vi "Simulated gated signals.vi"() -> ()   [LabVIEW 2022 SP3]
doc: "Performs real-time Joint Time Frequency Analysis (JTFA) using Point By Point STFT. The signal is simulated by a sine wave plus Gaussian noise."
uses:
  <vilib>/measure/mamon.llb/Waveform Peak Detection for N Chan.vi
  <vilib>/measure/NI_MAPro.lvlib
  <vilib>/gmath/NI_Gmath.lvlib
  <vilib>/Analysis/NI_AALBase.lvlib
panel:
  out "sampling frequency":dbl=16000.0
  out "BPM":dbl=260.6047910019081
  out "standard deviation":dbl=0.007320347822328487 format="%.4f"
  out "mean":dbl=0.23023367977744008 format="%.3f"
  out "Heart rates":dbl[](array[numeric])=[0.0, 0.23739526238057532, 0.21927218547308347, 0.22913219297822318, 0.2288319629419665, 0.2365367951133519]
  out "Waveform Graph 3":dynamicdata(graph)=[{"t0"=timestamp(0 s since 1904-01-01), "dt"=0.004, "Y"=array[365 elements], "attributes"=variant("NI_ChannelName"=variant(string "Filtered"))}]
  out "Array 4":i32[](array[numeric])=[1, 1, 1, 1, 1, 1, 1, 1, 1, 1, 0, 0, 0, 0, 0, 0, 0, 0, 1, 0, 0, 0, 0, 0, 0, 0, 0, 0, 0, 0, 0, 2, 0, 3, 4, 2, 5, 6, 3, 5, 7, 6, 7, 6, 6, 4, 5, 4, 6, 4, 4, 2, 3, 4, 2, 2, 1, 2, 1, 1, 1, 0, 0, 0, 0, 0, 0, 0, 0, 0, 0, 0, 0, 0, 0, 0, 0, 0, 0, 0, 0, 1, 1, 1, 1, 0, 0, 0, 1, 4, 2, 5, 4, 5, 4, 5, 3, 7, 5, 7, 5, 6, 5, 6, 5, 5, 5, 5, 6, 4, 2, 4, 2, 2, 2, 2, 1, 2, 1, 1, 1, 1, 1, 0, 0, 0, 0, 0, 1, 0, 1, 0, 0, 1, 0, 0, 0, 0, 0, 0, 0, 1, 0, 0, 1, 2, 2, 4, 6, 6, 6, 4, 8, 7, 5, 8, 5, 4, 5, 7, 6, 7, 5, 5, 5, 4, 4, 3, 3, 4, 3, 3, 1, 1, 1, 1, 1, 0, 1, 0, 0, 0, 0, 1, 0, 0, 0, 0, 1, 0, 0, 0, 0, 0, 0, 0, 0, 0, 1, 0, 0, 0, 3, 4, 4, 6, 6, 5, 6, 8, 8, 7, 6, 6, 7, 6, 6, 5, 7, 6, 6, 6, 5, 3, 4, 5, 3, 3, 2, 1, 1, 1, 1, 1, 0, 1, 0, 0, 1, 0, 0, 0, 0, 0, 0, 1, 0, 1, 0, 0, 1, 0, 1, 0, 1, 0, 1, 0, 1, 0, 2, 2, 3, 1, 4, 6, 5, 3, 5, 6, 4, 3, 3, 3, 3, 4, 3, 2, 2, 3, 4, 2, 2, 2, 2, 2, 2, 1, 1, 1, 1, 1, 1, 1, 1, 1, 1, 1, 1, 0, 0, 0, 1, 0, 0, 0, 0, 0, 0, 2, 0, 0, 0, 0, 0, 0, 1, 3, 3, 4, 5, 2, 4, 6, 4, 4, 5, 6, 6, 5, 6, 6, 6, 6, 6, 4, 5, 4, 2, 4, 3, 4, 2, 1, 1, 1, 1, 0, 1, 1, 1, 0, 0, 0, 1, 0, 0, 0, 0, 0, 0, 1, 0, 0, 1]
  out "Width 2":i32=365
  in  "time-freq config":cluster{"power of 2":bool, "Nyquist":bool}
  in  "Threshold":dbl=5.0
  in  "Width":i32=4
  in  "stop 2":bool
  out "Number of samples":i32=23336
  out "Extracted":dynamicdata(graph)=[{"t0"=timestamp(1.3140625000000001 s since 1904-01-01), "dt"=6.25e-05, "Y"=array[23336 elements], "attributes"=variant("NI_ChannelName"=variant(string "Dev1/ai0 (Extracted)"), "NI_ExpIsRelativeTime"=variant(bool TRUE), "NI_ExpStartTimeStamp"=variant(timestamp timestamp(3271175784.421062 s since 1904-01-01)), "NI_ExpTimeStamp"=variant(timestamp timestamp(3271175788.8760614 s since 1904-01-01)), "NI_ExpXDimension"=variant(string "t"), "NI_OriginalChannelName"=variant(string "Dev1/ai0"))}] caption="Signals"
  in  "process data":bool
  in  "time-freq sampling":cluster{"time steps":i32, "freq bins":i32}={"time steps"=64, "freq bins"=128} {"freq bins" format="%0.0f"}
  in  "window info":cluster{"type":u32, "window length":u32}={"type"=2, "window length"=128} {"window length" format="%0.0f"; "type" format="%0.0f"}
  out "Waveform Graph 2":waveform(dbl)(graph)={"t0"=timestamp(0 s since 1904-01-01), "dt"=0.004, "Y"=array[365 elements]}
  out "Locations":cluster{"Locations":dbl[]}[](array[cluster])=[{"Locations"=[49.01745339243051, 108.36626898757434, 163.1843153558452, 220.467363600401, 277.6753543358926, 336.8095531142306]}] {"Locations" format="%.2p"}
  out "Amplitudes":cluster{"Amplitudes":dbl[]}[](array[cluster])=[{"Amplitudes"=[82.38140614123277]}, {"Amplitudes"=[23.103240542422952]}, {"Amplitudes"=[179.84302922359947]}, {"Amplitudes"=[69.20602969118777]}, {"Amplitudes"=[166.80882400642417]}, {"Amplitudes"=[77.52276422393723]}, {"Amplitudes"=[21.4640593868428]}, {"Amplitudes"=[20.107049640024623]}, {"Amplitudes"=[8.747151960239117]}, {"Amplitudes"=[22.2070032831398]}, {"Amplitudes"=[]}, {"Amplitudes"=[]}, {"Amplitudes"=[]}, {"Amplitudes"=[]}, {"Amplitudes"=[]}, {"Amplitudes"=[]}, {"Amplitudes"=[]}, {"Amplitudes"=[]}, {"Amplitudes"=[5.038436740788092]}, {"Amplitudes"=[]}, {"Amplitudes"=[]}, {"Amplitudes"=[]}, {"Amplitudes"=[]}, {"Amplitudes"=[]}, {"Amplitudes"=[]}, {"Amplitudes"=[]}, {"Amplitudes"=[]}, {"Amplitudes"=[]}, {"Amplitudes"=[]}, {"Amplitudes"=[]}, {"Amplitudes"=[]}, {"Amplitudes"=[22.842667263708673, 6.3391147998422825]}, {"Amplitudes"=[]}, {"Amplitudes"=[24.87960791496652, 18.099361302359405, 11.032350413832436]}, {"Amplitudes"=[32.15025039562714, 13.922752510400683, 7.537223901883069, 8.901460877167851]}, {"Amplitudes"=[6.919633956075483, 6.805974509190123]}, {"Amplitudes"=[9.291208559626742, 9.83940570113674, 19.712031302498918, 10.262114635729274, 16.148451130689434]}, {"Amplitudes"=[58.61965660372665, 9.272847341081285, 10.229585203806352, 8.33485828928211, 8.53822283822932, 10.363752661085321]}, {"Amplitudes"=[32.99317191422573, 25.184044683933838, 6.176018204109812]}, {"Amplitudes"=[24.784936643849996, 11.180097278969077, 10.426571385559898, 9.147862049386452, 5.3056033973289445]}, {"Amplitudes"=[28.86732717209763, 57.63574400772855, 9.936407211583475, 15.352865769442293, 7.430357498420502, 9.113919835956231, 5.758941008482342]}, {"Amplitudes"=[30.501710958611454, 9.983123212214235, 49.565628988940404, 15.957520448688324, 5.142299425348082, 5.542245542198177]}, {"Amplitudes"=[13.584188049747981, 21.738357840547337, 21.353114728112995, 19.064944754501603, 12.767713772677945, 5.8155103082985375, 12.38997676581007]}, {"Amplitudes"=[19.17611366053601, 18.03811348206983, 21.946319425374636, 29.131558149158767, 7.854839251223176, 7.587917409227231]}, {"Amplitudes"=[26.251064738468205, 22.32439049471829, 13.733976720916365, 14.284625689843542, 11.06250138130756, 29.699723502437603]}, {"Amplitudes"=[13.92238514317977, 7.02343083135868, 95.53112318708045, 11.003700676197488]}, {"Amplitudes"=[75.27576626556457, 108.6469533115197, 46.189476972060085, 6.657679907425096, 6.508395743341386]}, {"Amplitudes"=[38.93368826176039, 22.453719389339394, 15.70774563803036, 25.85362047641387]}, {"Amplitudes"=[16.43990619327277, 11.31756210221035, 24.319042387903707, 22.55410151565015, 17.576151247289495, 6.909780980309922]}, {"Amplitudes"=[38.642716598694676, 68.69914689572425, 15.77436441173343, 17.57003043557135]}, {"Amplitudes"=[45.619636519793985, 66.77776746865493, 27.414381321266774, 10.378734791849856]}, {"Amplitudes"=[31.52012443340925, 9.419069673822978]}, {"Amplitudes"=[14.282507680413168, 30.083275487465478, 10.56411972040232]}, {"Amplitudes"=[17.52357745400949, 39.06632267195957, 67.90378041221246, 7.03859185888409]}, {"Amplitudes"=[38.22382741700391, 78.81409489667777]}, {"Amplitudes"=[99.66718914407029, 39.26256050528829]}, {"Amplitudes"=[121.01146302765554]}, {"Amplitudes"=[43.06727266056416, 14.211732733807018]}, {"Amplitudes"=[334.0636434809306]}, {"Amplitudes"=[197.95811877505346]}, {"Amplitudes"=[7.628663545669674]}, {"Amplitudes"=[]}, {"Amplitudes"=[]}, {"Amplitudes"=[]}, {"Amplitudes"=[]}, {"Amplitudes"=[]}, {"Amplitudes"=[]}, {"Amplitudes"=[]}, {"Amplitudes"=[]}, {"Amplitudes"=[]}, {"Amplitudes"=[]}, {"Amplitudes"=[]}, {"Amplitudes"=[]}, {"Amplitudes"=[]}, {"Amplitudes"=[]}, {"Amplitudes"=[]}, {"Amplitudes"=[]}, {"Amplitudes"=[]}, {"Amplitudes"=[]}, {"Amplitudes"=[]}, {"Amplitudes"=[]}, {"Amplitudes"=[38.02896888352999]}, {"Amplitudes"=[60.71594429484877]}, {"Amplitudes"=[77.864673975236]}, {"Amplitudes"=[86.75331398374871]}, {"Amplitudes"=[]}, {"Amplitudes"=[]}, {"Amplitudes"=[]}, {"Amplitudes"=[30.285694406280772]}, {"Amplitudes"=[6.70083506344839, 9.996184325043538, 13.161601140869823, 11.068127320638746]}, {"Amplitudes"=[12.179672839603471, 15.15864622255311]}, {"Amplitudes"=[6.757699919664426, 14.563558566945403, 30.0974793381078, 35.13852702699444, 11.82912775073785]}, {"Amplitudes"=[30.21628667420045, 37.19105776834435, 10.44811719015927, 5.979410571766171]}, {"Amplitudes"=[12.568666333491867, 10.525198573111078, 25.908754410806793, 23.480087021227384, 7.711006153248385]}, {"Amplitudes"=[8.069198985980876, 49.38285487269324, 16.54495588616374, 6.005677169490166]}, {"Amplitudes"=[9.974388294197606, 28.38980644929219, 12.125908243362064, 10.394406035302056, 12.273928645626906]}, {"Amplitudes"=[44.25850209386394, 45.36184860767733, 14.919613359784044]}, {"Amplitudes"=[25.551642802149477, 19.553635465036656, 47.25245815923574, 25.153362046593475, 14.160489368192284, 13.383198080728581, 15.616706212026298]}, {"Amplitudes"=[8.585910286384838, 49.15376283146787, 35.0730060764914, 19.924436039092853, 5.0061812311169795]}, {"Amplitudes"=[6.583257420688857, 6.2255192674828805, 45.69894868242657, 11.403330231694829, 23.57700544456967, 10.436565239964331, 11.383870447954372]}, {"Amplitudes"=[62.02127332764015, 33.96249128412671, 31.66759689025207, 23.0624840067356, 16.33642520284919]}, {"Amplitudes"=[34.415707375153936, 10.373696441976328, 26.156329918410478, 22.768141555256843, 10.750393432856006, 6.062207171974502]}, {"Amplitudes"=[32.48087650197277, 33.18602344776615, 17.890767174979935, 7.761315184410173, 5.7887068311030285]}, {"Amplitudes"=[37.083089931075314, 15.613396366499963, 12.051173949030618, 18.998380068120078, 5.577481300514407, 16.822493856755596]}, {"Amplitudes"=[116.412866314646, 47.39382629648723, 35.45067946475894, 8.848064961792382, 12.33559214796111]}, {"Amplitudes"=[36.55122432846308, 20.62731946396467, 19.524064296664893, 17.037236783177224, 12.75331545962354]}, {"Amplitudes"=[13.678435249173804, 17.977927437594456, 58.54736305377815, 37.905893287547244, 14.190662435858426]}, {"Amplitudes"=[19.7560860518155, 14.608744151622977, 14.997554396578456, 21.598462686694923, 6.803511160283876]}, {"Amplitudes"=[6.585864083905273, 16.35640196679662, 40.97026196636454, 5.74845196116436, 10.859839534328385, 26.432671751231265]}, {"Amplitudes"=[37.14491370258239, 8.786630443687102, 50.50402558068138, 6.9178735457692735]}, {"Amplitudes"=[43.03391314367019, 23.104668104550083]}, {"Amplitudes"=[19.23442411554904, 42.951474267999565, 8.326360458916051, 19.85487475354863]}, {"Amplitudes"=[67.38130875885368, 127.24575233366998]}, {"Amplitudes"=[230.59836703695711, 21.27374517334955]}, {"Amplitudes"=[117.60370625127554, 9.164920650883204]}, {"Amplitudes"=[34.48653974052241, 28.06721753602859]}, {"Amplitudes"=[97.08351402694935]}, {"Amplitudes"=[42.47704129034807, 11.196688692677348]}, {"Amplitudes"=[80.09104308548649]}, {"Amplitudes"=[17.024047125400102]}, {"Amplitudes"=[49.16287496060881]}, {"Amplitudes"=[37.874323635207055]}, {"Amplitudes"=[13.996901677633218]}, {"Amplitudes"=[]}, {"Amplitudes"=[]}, {"Amplitudes"=[]}, {"Amplitudes"=[]}, {"Amplitudes"=[]}, {"Amplitudes"=[21.059179416556383]}, {"Amplitudes"=[]}, {"Amplitudes"=[5.655247392917452]}, {"Amplitudes"=[]}, {"Amplitudes"=[]}, {"Amplitudes"=[7.566160612918716]}, {"Amplitudes"=[]}, {"Amplitudes"=[]}, {"Amplitudes"=[]}, {"Amplitudes"=[]}, {"Amplitudes"=[]}, {"Amplitudes"=[]}, {"Amplitudes"=[]}, {"Amplitudes"=[7.940747799708725]}, {"Amplitudes"=[]}, {"Amplitudes"=[]}, {"Amplitudes"=[171.89064010452762]}, {"Amplitudes"=[53.38985445160456, 47.20944180326978]}, {"Amplitudes"=[39.43321909539199, 41.42355004804408]}, {"Amplitudes"=[35.43003439390867, 39.79903190772515, 8.314447339982246, 5.522839392912958]}, {"Amplitudes"=[17.70458188715799, 22.27340772615113, 11.859423616096409, 16.196217369343895, 13.878592440001153, 9.367139271726463]}, {"Amplitudes"=[10.902753813737803, 51.224945091558666, 26.28363330510103, 12.775051212225032, 19.185592807108467, 16.064310141996202]}, {"Amplitudes"=[10.775132950480547, 9.837669766466332, 6.450044817928087, 40.14331590442509, 15.606677966367329, 5.604758984152606]}, {"Amplitudes"=[6.956894212125345, 36.49419940460505, 29.45502817761903, 8.942586285160438]}, {"Amplitudes"=[15.959514391389876, 18.853571112883863, 17.94415105779546, 38.525933539883226, 24.04328588184206, 21.273783492422787, 13.829695847414577, 7.0329830848447585]}, {"Amplitudes"=[19.739115058203684, 7.443389173941418, 59.547360360705206, 7.508154414957717, 7.263707742763704, 7.093406442203529, 13.645592171928815]}, {"Amplitudes"=[58.00433167997356, 66.44232976379686, 31.068545997989553, 7.732699625859007, 29.475986606683623]}, {"Amplitudes"=[20.029286291449644, 28.33111106014688, 8.409477614266663, 18.80578148132153, 21.171639700146116, 25.473492332663604, 7.755959491068256, 5.339663761530281]}, {"Amplitudes"=[48.57178655340573, 45.86566940589032, 33.80312552414865, 33.80004450551245, 5.5710069746768545]}, {"Amplitudes"=[33.80689208354685, 7.9078152784270115, 12.213787607759153, 8.29289788679703]}, {"Amplitudes"=[11.477744418191296, 50.28304189114041, 62.73404211139437, 9.263680695435566, 11.384540967823002]}, {"Amplitudes"=[20.993160472233647, 16.444118860252896, 16.553516223741497, 25.592202531125537, 5.470654244994138, 10.01144042489008, 9.484975090197048]}, {"Amplitudes"=[11.479156218631724, 14.712869975625633, 23.311470173881315, 30.955710724525687, 17.020590082910363, 26.38350872695788]}, {"Amplitudes"=[27.085772245284435, 11.746088084069942, 39.376986923391826, 24.5264042480838, 26.77428596744944, 5.6044046609893154, 5.298175841656865]}, {"Amplitudes"=[28.38274728899761, 76.88706276985069, 8.013736159658887, 8.38031009484177, 14.611102559246898]}, {"Amplitudes"=[76.77827122135417, 19.037720260357304, 9.60326338877064, 11.596331053222297, 12.442405338013234]}, {"Amplitudes"=[36.85058813068084, 48.469348137433265, 6.960250683572345, 17.964512808014693, 7.452668984994276]}, {"Amplitudes"=[17.45097214816472, 36.274815610259395, 7.190677788228538, 18.76892485635103]}, {"Amplitudes"=[60.84526604288865, 25.936192990356506, 43.43036376320756, 16.44188367868034]}, {"Amplitudes"=[18.39778665117683, 73.8231500979987, 22.207642893719008]}, {"Amplitudes"=[30.503574441126503, 15.987498475945522, 24.22199672355244]}, {"Amplitudes"=[46.736240717689924, 34.9927912752445, 18.712995867881926, 8.593473692159462]}, {"Amplitudes"=[24.95015968961785, 70.9578624318096, 23.31153075192986]}, {"Amplitudes"=[129.88897037632248, 19.359392264278593, 14.29879369556758]}, {"Amplitudes"=[52.42348108138743]}, {"Amplitudes"=[249.06110720379843]}, {"Amplitudes"=[191.33436863936132]}, {"Amplitudes"=[224.3389949048854]}, {"Amplitudes"=[50.621387641481356]}, {"Amplitudes"=[]}, {"Amplitudes"=[26.213300510084814]}, {"Amplitudes"=[]}, {"Amplitudes"=[]}, {"Amplitudes"=[]}, {"Amplitudes"=[]}, {"Amplitudes"=[7.327739677675397]}, {"Amplitudes"=[]}, {"Amplitudes"=[]}, {"Amplitudes"=[]}, {"Amplitudes"=[]}, {"Amplitudes"=[20.843287796685257]}, {"Amplitudes"=[]}, {"Amplitudes"=[]}, {"Amplitudes"=[]}, {"Amplitudes"=[]}, {"Amplitudes"=[]}, {"Amplitudes"=[]}, {"Amplitudes"=[]}, {"Amplitudes"=[]}, {"Amplitudes"=[]}, {"Amplitudes"=[7.387884548076854]}, {"Amplitudes"=[]}, {"Amplitudes"=[]}, {"Amplitudes"=[]}, {"Amplitudes"=[21.928584945420013, 36.678334521919744, 6.3634614463601595]}, {"Amplitudes"=[24.168064469562033, 59.46748182549027, 25.12585056357849, 9.25128990740101]}, {"Amplitudes"=[36.973845816800306, 38.41023801261688, 12.199245580540078, 20.848417096484578]}, {"Amplitudes"=[7.589284921506626, 37.10628507566227, 36.78179053718275, 19.153834405672583, 14.788215842131207, 31.497538241973427]}, {"Amplitudes"=[7.462862834423841, 33.64356982483671, 35.687193572807665, 10.914714968246365, 6.395307357205199, 7.481645977052394]}, {"Amplitudes"=[21.389333528673074, 30.65652762007901, 13.640171280184678, 38.00658119030499, 6.736822267190352]}, {"Amplitudes"=[30.874110552850833, 10.151323367710019, 13.407506388034585, 15.657040012186263, 24.948348238396658, 5.553012250177308]}, {"Amplitudes"=[12.638697518333654, 21.21924704328737, 20.04632407096911, 10.939049908723215, 9.636104102619631, 6.1924783838874005, 6.158926380111476, 5.225816391256243]}, {"Amplitudes"=[14.395293156948524, 86.02588457815224, 23.624264443146032, 25.472728212443773, 6.090105619826654, 13.574769357585836, 7.545745626953435, 8.47833478533895]}, {"Amplitudes"=[10.057184760704034, 13.700392719608312, 13.295119125901904, 17.646676773137532, 12.8355956282058, 5.432264220622043, 6.639568708824927]}, {"Amplitudes"=[12.668743392842478, 16.369950467735308, 17.98653933948661, 7.593794311076839, 8.20927268702362, 6.498272033238524]}, {"Amplitudes"=[14.031400641894509, 28.344208540059995, 48.82277302182409, 21.61919187363569, 17.54071548303219, 12.512146355785518]}, {"Amplitudes"=[66.82348885694685, 10.543085108407302, 29.82388792286026, 15.930922112126945, 9.358963610667939, 5.722002653071298, 7.54226261694091]}, {"Amplitudes"=[46.884270147985774, 47.30955825337601, 12.137346047861453, 17.241069172388947, 6.727790715965158, 8.941716613328515]}, {"Amplitudes"=[15.745933005132843, 27.019142762223254, 26.80018633540539, 46.32040002305749, 10.853667553214647, 12.19027891958808]}, {"Amplitudes"=[12.801454246943333, 44.66850079977029, 25.47489461369436, 28.725762021631784, 5.5246298475093605]}, {"Amplitudes"=[23.710778045458547, 32.09565954363097, 9.759838650281145, 13.96227854351386, 22.839370068639635, 8.616436223748197, 16.601250003868067]}, {"Amplitudes"=[21.091792243972556, 80.61966420696207, 10.161102286135073, 26.325545390510076, 12.431990072819296, 15.297216040962423]}, {"Amplitudes"=[14.169342013145188, 68.48741584667661, 20.287271047901033, 10.45724066171925, 22.304048328735295, 16.279664127845336]}, {"Amplitudes"=[23.698319669770985, 18.53830082049265, 16.963482366871055, 26.094611347090325, 19.065292954754586, 26.026458475425862]}, {"Amplitudes"=[8.8551740920852, 54.97624726567635, 29.100032383551742, 38.31610896219175, 21.06941321612808]}, {"Amplitudes"=[32.201459426893976, 6.237302033154788, 12.59854517839782]}, {"Amplitudes"=[28.022223819932623, 40.25413349929261, 8.16546400342377, 26.900148863252173]}, {"Amplitudes"=[36.16132943102215, 53.805081332739945, 37.13126740271426, 27.063843599868864, 11.077328288512884]}, {"Amplitudes"=[98.91263436778961, 18.604487901013343, 11.887150221932503]}, {"Amplitudes"=[14.605725900968638, 25.58205471891051, 17.939415172165607]}, {"Amplitudes"=[68.97917326599013, 34.87106937537459]}, {"Amplitudes"=[171.4708356256902]}, {"Amplitudes"=[175.83627487125722]}, {"Amplitudes"=[56.15561136805608]}, {"Amplitudes"=[5.5645477697375885]}, {"Amplitudes"=[40.841000614624484]}, {"Amplitudes"=[]}, {"Amplitudes"=[34.20994360835842]}, {"Amplitudes"=[]}, {"Amplitudes"=[]}, {"Amplitudes"=[5.403980623079512]}, {"Amplitudes"=[]}, {"Amplitudes"=[]}, {"Amplitudes"=[]}, {"Amplitudes"=[]}, {"Amplitudes"=[]}, {"Amplitudes"=[]}, {"Amplitudes"=[13.175507639769348]}, {"Amplitudes"=[]}, {"Amplitudes"=[14.318195074759418]}, {"Amplitudes"=[]}, {"Amplitudes"=[]}, {"Amplitudes"=[8.415802727161436]}, {"Amplitudes"=[]}, {"Amplitudes"=[37.43508642182159]}, {"Amplitudes"=[]}, {"Amplitudes"=[40.94982541525543]}, {"Amplitudes"=[]}, {"Amplitudes"=[74.40151251115563]}, {"Amplitudes"=[]}, {"Amplitudes"=[80.2212185190783]}, {"Amplitudes"=[]}, {"Amplitudes"=[46.14870460546982, 8.203231597370932]}, {"Amplitudes"=[44.96986333451507, 31.0173959313927]}, {"Amplitudes"=[47.20729662527929, 16.658170670106752, 13.805614358779534]}, {"Amplitudes"=[14.242109835465094]}, {"Amplitudes"=[16.357427091265095, 27.678687240186143, 14.190433241707423, 5.970546566655532]}, {"Amplitudes"=[7.338450447251885, 27.53965839209764, 9.372772208808492, 16.977143482657908, 25.326385278892825, 12.254726972920094]}, {"Amplitudes"=[13.662555584641327, 10.072853844691418, 15.1471251401094, 34.609858994690505, 15.150354096091851]}, {"Amplitudes"=[33.37989835067148, 22.084862887613067, 8.638940338410627]}, {"Amplitudes"=[11.122108485372156, 9.810037971771518, 17.030740276217294, 6.776864726572519, 8.280175360361017]}, {"Amplitudes"=[26.211060153758247, 36.35955379899989, 10.726362279232289, 17.189819578120282, 14.514506995872479, 26.052771948840093]}, {"Amplitudes"=[13.607242544347233, 5.778340762637316, 10.040343122054113, 19.50136011101791]}, {"Amplitudes"=[20.475751050063796, 17.684066349955152, 8.552349753403005]}, {"Amplitudes"=[23.738980108843975, 8.418711614882344, 9.84430997025031]}, {"Amplitudes"=[9.46821524381136, 10.072642754608044, 14.323339724886976]}, {"Amplitudes"=[13.587221258378793, 7.242832508077184, 8.223942310063887]}, {"Amplitudes"=[38.53515156615356, 6.316620777874599, 7.118552845128106, 12.582977985255408]}, {"Amplitudes"=[8.416483079417631, 5.762969748973174, 7.793031192256171]}, {"Amplitudes"=[10.494851008067169, 5.292092808905673]}, {"Amplitudes"=[5.450904392073333, 11.957166360585985]}, {"Amplitudes"=[6.586888755493399, 5.315357285083652, 5.517723695652094]}, {"Amplitudes"=[19.49486335582361, 5.970534172263876, 5.846414330033691, 16.852040354876326]}, {"Amplitudes"=[7.3379383793021455, 8.369071846807326]}, {"Amplitudes"=[16.392780314808952, 5.0801345088275625]}, {"Amplitudes"=[7.258450608294382, 11.692002338386105]}, {"Amplitudes"=[10.63184587196843, 18.567304548275864]}, {"Amplitudes"=[30.3609172581837, 7.400709984781025]}, {"Amplitudes"=[13.38322083489419, 15.352570266967962]}, {"Amplitudes"=[42.31891944491651]}, {"Amplitudes"=[67.81202236395082]}, {"Amplitudes"=[65.27036998165693]}, {"Amplitudes"=[28.455418795098577]}, {"Amplitudes"=[5.148448044439733]}, {"Amplitudes"=[8.758151498242388]}, {"Amplitudes"=[56.12915877934294]}, {"Amplitudes"=[121.01673791026457]}, {"Amplitudes"=[102.32173969545939]}, {"Amplitudes"=[133.96620399340688]}, {"Amplitudes"=[191.43971005308586]}, {"Amplitudes"=[115.97727310627029]}, {"Amplitudes"=[]}, {"Amplitudes"=[]}, {"Amplitudes"=[]}, {"Amplitudes"=[8.4807715713379]}, {"Amplitudes"=[]}, {"Amplitudes"=[]}, {"Amplitudes"=[]}, {"Amplitudes"=[]}, {"Amplitudes"=[]}, {"Amplitudes"=[]}, {"Amplitudes"=[5.667430954402727, 5.204097018640564]}, {"Amplitudes"=[]}, {"Amplitudes"=[]}, {"Amplitudes"=[]}, {"Amplitudes"=[]}, {"Amplitudes"=[]}, {"Amplitudes"=[]}, {"Amplitudes"=[229.37835261204367]}, {"Amplitudes"=[112.73062783307276, 68.11323938327236, 37.64581689964294]}, {"Amplitudes"=[31.91448396753468, 12.743891515209286, 23.674439565274643]}, {"Amplitudes"=[17.598432765028797, 74.94489884709694, 11.64986705427759, 11.47288421684143]}, {"Amplitudes"=[19.77976789822392, 40.4683311943491, 13.209832687017466, 24.2708060506737, 12.67480033911827]}, {"Amplitudes"=[136.5993255217836, 6.981426404432122]}, {"Amplitudes"=[65.66768714015453, 10.97678190363755, 7.276200536104776, 22.967689977543138]}, {"Amplitudes"=[8.02714483414711, 38.32427098468889, 13.848458769580839, 11.300020220412902, 16.052146962561565, 9.57398992631342]}, {"Amplitudes"=[15.518984866284212, 55.77255374707614, 10.507840019292582, 6.7850630079557686]}, {"Amplitudes"=[61.24369432344984, 14.008597463561475, 33.340308419327144, 25.58370031623873]}, {"Amplitudes"=[9.358323852228244, 36.00586733114804, 30.928246842105956, 35.26916269215111, 11.465928274825117]}, {"Amplitudes"=[25.63503577035782, 13.136272143472837, 36.90489778392109, 25.402463584009862, 20.627052733975678, 42.18164750473402]}, {"Amplitudes"=[24.630017382827795, 12.111619022839395, 22.677994530155704, 14.612743883029296, 10.095187523605729, 5.963974538221233]}, {"Amplitudes"=[37.665785897232894, 29.831847747635713, 43.908419186213806, 5.0932517146045235, 10.200846665881993]}, {"Amplitudes"=[36.42689318768818, 23.140285919433335, 33.73001978776403, 13.524011268910334, 21.56051594700629, 5.217110422805082]}, {"Amplitudes"=[17.573307222249777, 16.78081400523589, 48.5528828217628, 9.377670815281228, 9.593514528244501, 9.483828244483542]}, {"Amplitudes"=[16.415903374849897, 66.89623662563456, 7.879349232546521, 12.373959468734858, 7.522539528899703, 6.233440351832409]}, {"Amplitudes"=[16.47626563966333, 29.323905749676268, 36.32240827687618, 23.618367585040716, 10.540950305417022, 12.599190388357915]}, {"Amplitudes"=[12.635140258148196, 76.44975556381019, 63.39014639018582, 19.282629304642608, 6.819369115120635, 17.161035874757726]}, {"Amplitudes"=[51.03316435811473, 62.34818594593384, 10.788328995748838, 27.818378060643813]}, {"Amplitudes"=[25.685344106378135, 36.37829744531831, 31.105805534380053, 38.62375332094815, 8.381615322955206]}, {"Amplitudes"=[12.384553100143568, 12.16475381157859, 38.42070546138646, 25.285956275924352]}, {"Amplitudes"=[17.80350267098267, 37.66518397602322]}, {"Amplitudes"=[34.137704498819915, 15.246341812059939, 7.92787426368764, 24.584339379889688]}, {"Amplitudes"=[17.978350380256938, 47.33048385456938, 22.427713441573935]}, {"Amplitudes"=[39.68402621189873, 63.58968177708207, 38.11932882880105, 10.453711151395416]}, {"Amplitudes"=[99.38904014049761, 78.06923340571915]}, {"Amplitudes"=[60.91953840534908]}, {"Amplitudes"=[43.11761031194111]}, {"Amplitudes"=[119.80015356353208]}, {"Amplitudes"=[83.76358861166717]}, {"Amplitudes"=[]}, {"Amplitudes"=[79.76657397732446]}, {"Amplitudes"=[46.08892245151188]}, {"Amplitudes"=[29.59462992950242]}, {"Amplitudes"=[]}, {"Amplitudes"=[]}, {"Amplitudes"=[]}, {"Amplitudes"=[6.944567466962198]}, {"Amplitudes"=[]}, {"Amplitudes"=[]}, {"Amplitudes"=[]}, {"Amplitudes"=[]}, {"Amplitudes"=[]}, {"Amplitudes"=[]}, {"Amplitudes"=[14.25367943743587]}, {"Amplitudes"=[]}, {"Amplitudes"=[]}, {"Amplitudes"=[5.297319752195488]}] {"Amplitudes" format="%.2p"}
  out "# peaks found":i32[](array[numeric])=[1, 1, 1, 1, 1, 1, 1, 1, 1, 1, 0, 0, 0, 0, 0, 0, 0, 0, 1, 0, 0, 0, 0, 0, 0, 0, 0, 0, 0, 0, 0, 2, 0, 3, 4, 2, 5, 6, 3, 5, 7, 6, 7, 6, 6, 4, 5, 4, 6, 4, 4, 2, 3, 4, 2, 2, 1, 2, 1, 1, 1, 0, 0, 0, 0, 0, 0, 0, 0, 0, 0, 0, 0, 0, 0, 0, 0, 0, 0, 0, 0, 1, 1, 1, 1, 0, 0, 0, 1, 4, 2, 5, 4, 5, 4, 5, 3, 7, 5, 7, 5, 6, 5, 6, 5, 5, 5, 5, 6, 4, 2, 4, 2, 2, 2, 2, 1, 2, 1, 1, 1, 1, 1, 0, 0, 0, 0, 0, 1, 0, 1, 0, 0, 1, 0, 0, 0, 0, 0, 0, 0, 1, 0, 0, 1, 2, 2, 4, 6, 6, 6, 4, 8, 7, 5, 8, 5, 4, 5, 7, 6, 7, 5, 5, 5, 4, 4, 3, 3, 4, 3, 3, 1, 1, 1, 1, 1, 0, 1, 0, 0, 0, 0, 1, 0, 0, 0, 0, 1, 0, 0, 0, 0, 0, 0, 0, 0, 0, 1, 0, 0, 0, 3, 4, 4, 6, 6, 5, 6, 8, 8, 7, 6, 6, 7, 6, 6, 5, 7, 6, 6, 6, 5, 3, 4, 5, 3, 3, 2, 1, 1, 1, 1, 1, 0, 1, 0, 0, 1, 0, 0, 0, 0, 0, 0, 1, 0, 1, 0, 0, 1, 0, 1, 0, 1, 0, 1, 0, 1, 0, 2, 2, 3, 1, 4, 6, 5, 3, 5, 6, 4, 3, 3, 3, 3, 4, 3, 2, 2, 3, 4, 2, 2, 2, 2, 2, 2, 1, 1, 1, 1, 1, 1, 1, 1, 1, 1, 1, 1, 0, 0, 0, 1, 0, 0, 0, 0, 0, 0, 2, 0, 0, 0, 0, 0, 0, 1, 3, 3, 4, 5, 2, 4, 6, 4, 4, 5, 6, 6, 5, 6, 6, 6, 6, 6, 4, 5, 4, 2, 4, 3, 4, 2, 1, 1, 1, 1, 0, 1, 1, 1, 0, 0, 0, 1, 0, 0, 0, 0, 0, 0, 1, 0, 0, 1]
  out "Waveform Graph":dbl[](graph)=[17.836961991222946, 25.972936749911703, 7.943446483303552, 1.119503839835049, 0.7567421181239652, 7.168605720967425, 2.6514612003802998, 12.095482095719882, 7.320603997298466, 28.900786577261744, 28.616852086518776, 6.074795024837742, 11.023718833207578, 5.637421962434986, 0.6823366730399569, 0.907038579172145, 0.0075337053383707445, 1.1151801728675306, 2.948769091038062, 3.5533711252423115, 2.6428909195292016, 0.6991948791936987, 0.19364562661412105, 0.17899974987650524, 0.01610536979227146, 0.01883749348215313, 0.02557718744392, 0.050922535457355325, 0.03320065024063828, 0.005134247822773508, 0.002433910187436692, 0.0006444584084756639, 0.0004757436776852226, 0.001632848348371804, 0.0005183008552724987, 0.00018391097488622797, 0.0019942134949158625, 0.0002911654712398335, 0.0011448043490207428, 0.00026720684489327885, 0.00036609432398689365, 0.00037161025668843036, 0.0003024117565315067, 0.0009074817409475442, 9.63152901033982e-05, 0.00038047972784880914, 0.0008836372765696738, 0.0005241853156929144, 8.216937330578516e-05, 0.0006503020932542836, 0.00014365144060756433, 0.0003765563779985365, 0.0005207408463393673, 0.0003514652755409058, 0.00017199291132504287, 0.0008358385916806878, 6.592850004714467e-05, 0.0004060697824099824, 0.00037638225881807616, 0.000592724690944733, 0.0002831628985588985, 0.00028585924504815165, 0.0008137998097228686, 0.0013674269255811952, 7.843516963545003e-06]
  out "Array 3":dbl[][](array[numeric])
  out "Array 2":i32[](array[numeric])=[365, 65]
  out "Doppler signal":dynamicdata(graph)=[{"t0"=timestamp(0 s since 1904-01-01), "dt"=6.25e-05, "Y"=array[50000 elements], "attributes"=variant("NI_ChannelName"=variant(string "Dev1/ai0"), "NI_ExpIsRelativeTime"=variant(bool TRUE), "NI_ExpStartTimeStamp"=variant(timestamp timestamp(3271175784.421062 s since 1904-01-01)), "NI_ExpTimeStamp"=variant(timestamp timestamp(3271175787.561999 s since 1904-01-01)), "NI_ExpXDimension"=variant(string "t"))}] caption="Signals"
  out "Moving STFT":dbl[][](graph)
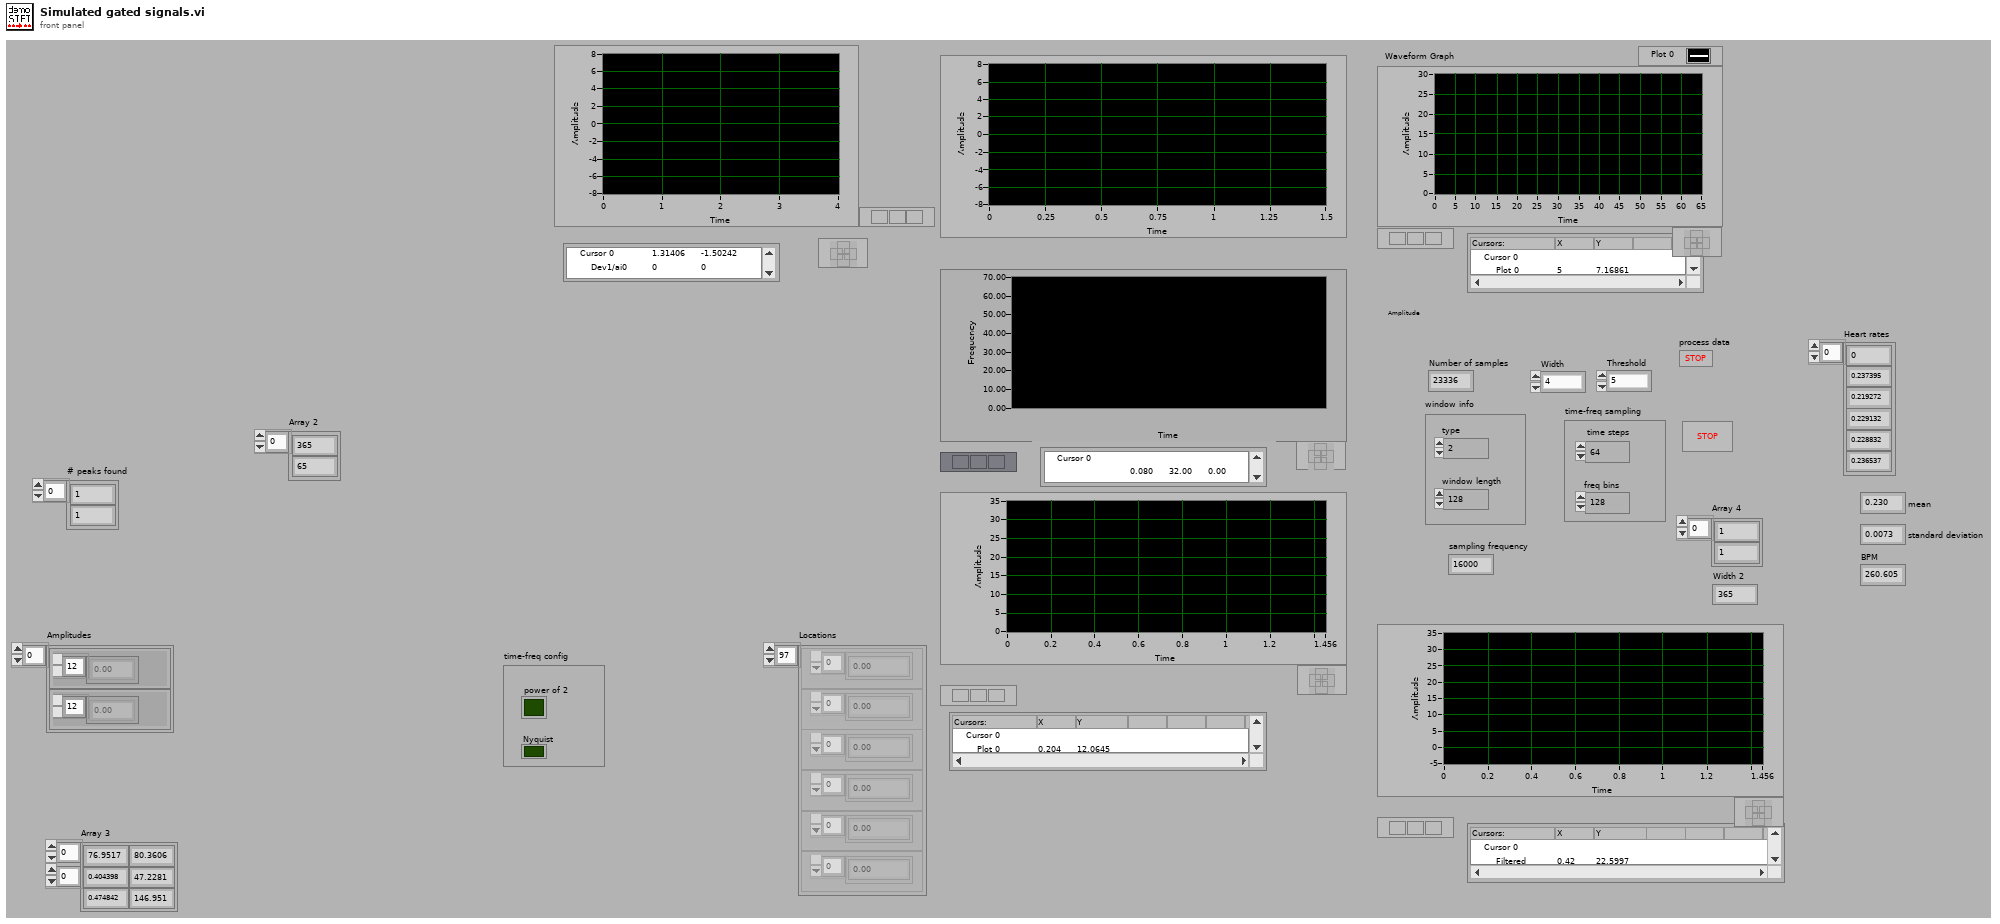
[diagram p1: front panel]
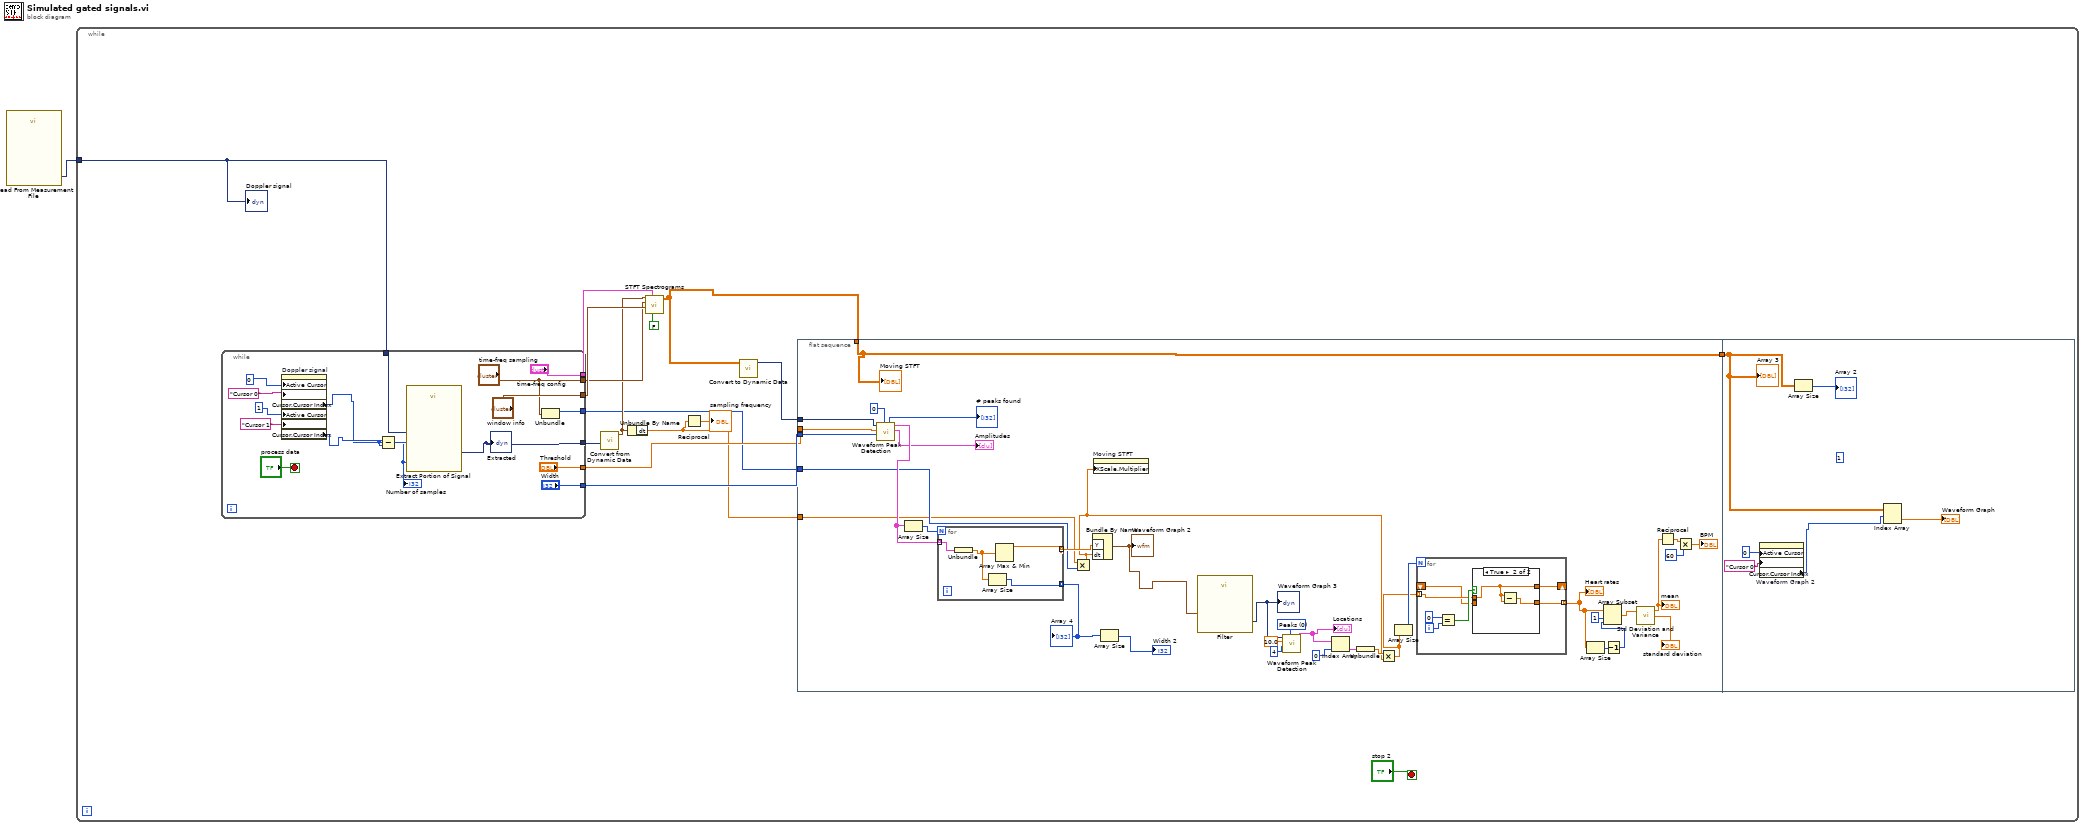
[diagram p0: block diagram]
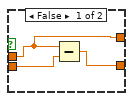
[diagram p2: hidden frame]
diagram:
  n1 = call "Read From Measurement File"() -> ("Signals"=w1:dynamicdata)  [unwired: 4 in, 7 out]
  n2 = while {
    tunnel: w1 -> [w13]
    stop <- "stop 2" stop-if-true
    n3 = while {
      tunnel: w13 -> [w88]
      tunnel: [w80] -> w16
      tunnel: ["window info"] -> w15
      tunnel: ["time-freq sampling"] -> w14
      tunnel: ["Threshold"] -> w7
      tunnel: ["Width"] -> w8
      tunnel: ["time-freq config"] -> w11
      tunnel: [w76] -> w4
      stop <- "process data" stop-if-true
      n4 = property on="Doppler signal" class="WFGraph (strict)"("Active Cursor"=0, "Cursor.Cursor Name"="Cursor 0", "Active Cursor"=1, "Cursor.Cursor Name"="Cursor 1") -> ("Cursor.Cursor Index"=w86:i32, "Cursor.Cursor Index"=w87:i32)  [unwired: 2 in, 2 out]
      n5 = Subtract(x=w87, y=w86) -> (x-y=w85:i32)
      "Number of samples" <- w85
      n6 = call "Extract Portion of Signal"("Samples"=w85, "Begin Sample"=w86, "Signals"=w88) -> ("Section"=w80:dynamicdata)  [unwired: 1 in, 7 out]
      "Extracted" <- w80
      n7 = Unbundle("time-freq sampling") -> ("time steps"=w76:i32)  [unwired: 1 out]
    }
    n8 = call "Convert from Dynamic Data"("Dynamic Data Type"=w16) -> ("Waveform"=w10:waveform(dbl))  [unwired: 1 in, 2 out]
    n9 = Unbundle By Name(w10) -> ("dt"=w3:dbl)
    n10 = call <vilib>:"STFT Spectrograms.vi"("energy conservation?"=FALSE, "time-freq config"=w11, "window info"=w15, "time-freq sampling info"=w14, "X"=w10) -> ("STFT Spectrogram {X}"=w6:dbl[][])  [unwired: 1 in, 5 out]
    n11 = Reciprocal(x=w3) -> (1/x=→"sampling frequency":dbl)
    n12 = call "Convert to Dynamic Data"("2D Array"=w6) -> ("Dynamic Data Type"=w9:dynamicdata)  [unwired: 3 out]
    n13 = flat-sequence {
      tunnel: w9 -> [w41]
      tunnel: w8 -> [w46]
      tunnel: w7 -> [w45]
      tunnel: w6 -> [w40]
      tunnel: [w40] -> w5
      tunnel: w4 -> [w43]
      tunnel: w3 -> [w42]
      tunnel: w5 -> [w75]
      frame #0 {
        w35 = u16 0 items=["Peaks", "Valleys"] ("peaks/valleys")
        n14 = call-poly <vilib>:"Waveform Peak Detection.vi"("peaks/valleys"=u32 0 ("milliseconds to wait"), "width"=w46, "threshold"=w45, "Signals In"=w41) -> ("Amplitudes"=→"Amplitudes":cluster{"Amplitudes":dbl[]}[], "Locations"=w50:cluster{"Locations":dbl[]}[], "# found"=→"# peaks found":i32[])  [unwired: 3 in, 2 out]
        n15 = Array Size(array=w50) -> (size(s)=w51:i32)
        n16 = for {
          N: w51 -> [_]
          tunnel: w50 -> [w69] mode=indexing
          tunnel: [w68] -> w44 mode=indexing
          tunnel: [w66] -> w52 mode=indexing
          n17 = Unbundle(w69) -> ("Locations"=w67:dbl[])
          n18 = Array Size(array=w67) -> (size(s)=w66:i32)
          n19 = Array Max & Min(array=w67) -> (max value=w68:dbl)  [unwired: 3 out]
        }
        "Array 4" <- w52
        n20 = Multiply(x=w42, y=w43) -> (x*y=w30:dbl)
        n21 = Bundle By Name("Y"=w44, "dt"=w30) -> (w39:waveform(dbl))  [unwired: 1 out]
        "Waveform Graph 2" <- w39
        n22 = property on="Moving STFT" class="IntGraph (strict)"("XScale.Multiplier"=w30) -> ()  [unwired: 2 in, 2 out]
        n23 = Array Size(array=w52) -> (size(s)=→"Width 2":i32)
        n24 = call "Filter"("Signal"=w39) -> ("Filtered Signal"=w38:dynamicdata)  [unwired: 2 in, 8 out]
        "Waveform Graph 3" <- w38
        n25 = call-poly <vilib>:"Waveform Peak Detection.vi"("peaks/valleys"=w35, "width"=4, "threshold"=10.0, "Signals In"=w38) -> ("Locations"=w34:cluster{"Locations":dbl[]}[])  [unwired: 3 in, 4 out]
        "Locations" <- w34
        n26 = Index Array(array=w34, index=0 ("width")) -> (element=w32:cluster{"Locations":dbl[]})
        n27 = Unbundle(w32) -> ("Locations"=w31:dbl[])
        n28 = Multiply(x=w31, y=w30) -> (x*y=w28:dbl[])
        n29 = Array Size(array=w28) -> (size(s)=w29:i32)
        n30 = for {
          N: w29 -> [_]
          tunnel: w28 -> [w57] mode=indexing
          shift-right: [w55] -> _
          shift-left: _ -> [w56]
          tunnel: [w54] -> w25 mode=indexing
          i -> [w60]
          n31 = Equal?(x=0, y=w60) -> (x = y?=w58:bool)
          n32 = case shown="True" w58 {
            tunnel: w57 -> [w62 w65]
            tunnel: [w62 w65] -> w55
            tunnel: w56 -> [w63 _]
            tunnel: [w61 w64] -> w54
            frame False {
              n33 = Subtract(x=w62, y=w63) -> (x-y=w61:dbl)
            }
            frame True {
              n34 = Subtract(x=w65, y=w65) -> (x-y=w64:dbl)
            }
          }
        }
        "Heart rates" <- w25
        n35 = Array Size(array=w25) -> (size(s)=w22:i32)
        n36 = Decrement(x=w22) -> (x-1=w24:i32)
        n37 = Array Subset(array=w25, index=1, length=w24) -> (w26:dbl[])
        n38 = call <vilib>:"Std Deviation and Variance.vi"("X"=w26) -> ("mean"=w21:dbl, "standard deviation"=→"standard deviation":dbl)  [unwired: 1 in, 1 out]
        "mean" <- w21
        n39 = Reciprocal(x=w21) -> (1/x=w20:dbl)
        n40 = Multiply(x=w20, y=60 ("index")) -> (x*y=→"BPM":dbl)
        "Moving STFT" <- w40
      }
      frame #1 {
        (unwired) u32 1 ("milliseconds to wait")
        n41 = property on="Waveform Graph 2" class="WFGraph (strict)"("Active Cursor"=0, "Cursor.Cursor Name"="Cursor 0") -> ("Cursor.Cursor Index"=w70:i32)  [unwired: 2 in, 2 out]
        n42 = Array Size(array=w75) -> (size(s)=→"Array 2":i32[])
        n43 = Index Array(array=w75, index (row)=w70) -> (element=→"Waveform Graph":dbl[])  [unwired: 1 in]
        "Array 3" <- w75
      }
    }
    "Doppler signal" <- w13
  }
